vi "update_param_expSD.vi"(3 "cluster in":T1={"Kinetics"=[], "Spectrum"=[], "Experiments groups"=[], "GRAPH EXPERIMENTAL DATA"=[], "error out"={"status"=FALSE, "code"=0, "source"=""}, "group"=0, "exp selected"=0, "# exp"=0, "kinetics plot names"=[], "spectra plot names"=[], "FromToWave"={"FromWave"=0.0, "ToWave"=0.0}, "Laser shutter task"="", "Accelerator task"="", "Motor task"="", "GRAPH EXPERIMENTAL DATA ref"=refnum, "timedelays"=[0.0, 0.0, 0.0, 0.0, 0.0, 0.0, 0.0, 0.06019061100911815, 0.0521779104562645, 0.045231877429679615, 0.03921051490799832, 0.033990728811568754, 0.029465811603150715, 0.025543260876973825, 0.02214288834180205, 0.01919518054014414, 0.016639877791965713, 0.014424742312398925, 0.012504490320209958, 0.010839866306230088, 0.009396840537117498, 0.008145913389103785, 0.00706151229029317, 0.006121468943269439, 0.005306566140927374, 0.004600144911132549, 0.003987763959109073, 0.0034569044455719407, 0.00299671406541447, 0.0025977851951783253, 0.0022519625739982996, 0.00195217658646366, 0.0016922987392150965, 0.0014670163768006634, 0.0012717240756200802, 0.0011024294957352762, 0.0009556717658856477, 0.0008284507332614981, 0.0007181656316962257, 0.0006225619144775864, 0.0005396851648867825, 0.00046784114226338394, 0.0004055611468220084, 0.0003515719951773376, 0.00030476999279031153, 0.00026419837125694315, 0.00022902772919263772, 0.0001985390768670671, 0.0001721091379728629, 0.00014919760805372974, 0.00012933610911736794], "wavelengths"=[0.0, 0.0, 0.0, 0.0, 0.0, 0.0, 0.0, 0.06019061100911815, 0.0521779104562645, 0.045231877429679615, 0.03921051490799832, 0.033990728811568754, 0.029465811603150715, 0.025543260876973825, 0.02214288834180205, 0.01919518054014414, 0.016639877791965713, 0.014424742312398925, 0.012504490320209958, 0.010839866306230088, 0.009396840537117498, 0.008145913389103785, 0.00706151229029317, 0.006121468943269439, 0.005306566140927374, 0.004600144911132549, 0.003987763959109073, 0.0034569044455719407, 0.00299671406541447, 0.0025977851951783253, 0.0022519625739982996, 0.00195217658646366, 0.0016922987392150965, 0.0014670163768006634, 0.0012717240756200802, 0.0011024294957352762, 0.0009556717658856477, 0.0008284507332614981, 0.0007181656316962257, 0.0006225619144775864, 0.0005396851648867825, 0.00046784114226338394, 0.0004055611468220084, 0.0003515719951773376, 0.00030476999279031153, 0.00026419837125694315, 0.00022902772919263772, 0.0001985390768670671, 0.0001721091379728629, 0.00014919760805372974, 0.00012933610911736794], "Experiment"=refnum, "Commentaires exp"=refnum, "FromToDelay"={"FromDelay"=0.0, "ToDelay"=0.0}}) -> (5 "Real delay time, ps":dbl=3790.0, 6 "numberpoints, ps":i32, 7 "deltaTlast":dbl, 8 "# current":i32, 9 "Delay0,ps":dbl=-200.0, 10 "cluster out":T1={"Kinetics"=[], "Spectrum"=[], "Experiments groups"=[], "GRAPH EXPERIMENTAL DATA"=[], "error out"={"status"=FALSE, "code"=0, "source"=""}, "group"=0, "exp selected"=0, "# exp"=0, "kinetics plot names"=[], "spectra plot names"=[], "FromToWave"={"FromWave"=0.0, "ToWave"=0.0}, "Laser shutter task"="", "Accelerator task"="", "Motor task"="", "GRAPH EXPERIMENTAL DATA ref"=refnum, "timedelays"=[0.0, 0.0, 0.0, 0.0, 0.0, 0.0, 0.0, 0.06019061100911815, 0.0521779104562645, 0.045231877429679615, 0.03921051490799832, 0.033990728811568754, 0.029465811603150715, 0.025543260876973825, 0.02214288834180205, 0.01919518054014414, 0.016639877791965713, 0.014424742312398925, 0.012504490320209958, 0.010839866306230088, 0.009396840537117498, 0.008145913389103785, 0.00706151229029317, 0.006121468943269439, 0.005306566140927374, 0.004600144911132549, 0.003987763959109073, 0.0034569044455719407, 0.00299671406541447, 0.0025977851951783253, 0.0022519625739982996, 0.00195217658646366, 0.0016922987392150965, 0.0014670163768006634, 0.0012717240756200802, 0.0011024294957352762, 0.0009556717658856477, 0.0008284507332614981, 0.0007181656316962257, 0.0006225619144775864, 0.0005396851648867825, 0.00046784114226338394, 0.0004055611468220084, 0.0003515719951773376, 0.00030476999279031153, 0.00026419837125694315, 0.00022902772919263772, 0.0001985390768670671, 0.0001721091379728629, 0.00014919760805372974, 0.00012933610911736794], "wavelengths"=[0.0, 0.0, 0.0, 0.0, 0.0, 0.0, 0.0, 0.06019061100911815, 0.0521779104562645, 0.045231877429679615, 0.03921051490799832, 0.033990728811568754, 0.029465811603150715, 0.025543260876973825, 0.02214288834180205, 0.01919518054014414, 0.016639877791965713, 0.014424742312398925, 0.012504490320209958, 0.010839866306230088, 0.009396840537117498, 0.008145913389103785, 0.00706151229029317, 0.006121468943269439, 0.005306566140927374, 0.004600144911132549, 0.003987763959109073, 0.0034569044455719407, 0.00299671406541447, 0.0025977851951783253, 0.0022519625739982996, 0.00195217658646366, 0.0016922987392150965, 0.0014670163768006634, 0.0012717240756200802, 0.0011024294957352762, 0.0009556717658856477, 0.0008284507332614981, 0.0007181656316962257, 0.0006225619144775864, 0.0005396851648867825, 0.00046784114226338394, 0.0004055611468220084, 0.0003515719951773376, 0.00030476999279031153, 0.00026419837125694315, 0.00022902772919263772, 0.0001985390768670671, 0.0001721091379728629, 0.00014919760805372974, 0.00012933610911736794], "Experiment"=refnum, "Commentaires exp"=refnum, "FromToDelay"={"FromDelay"=0.0, "ToDelay"=0.0}})   [LabVIEW 2015]
uses:
  controls/control-cluster.ctl
  Classes/Experiments_group.lvclass
  Classes/Experiment.lvclass
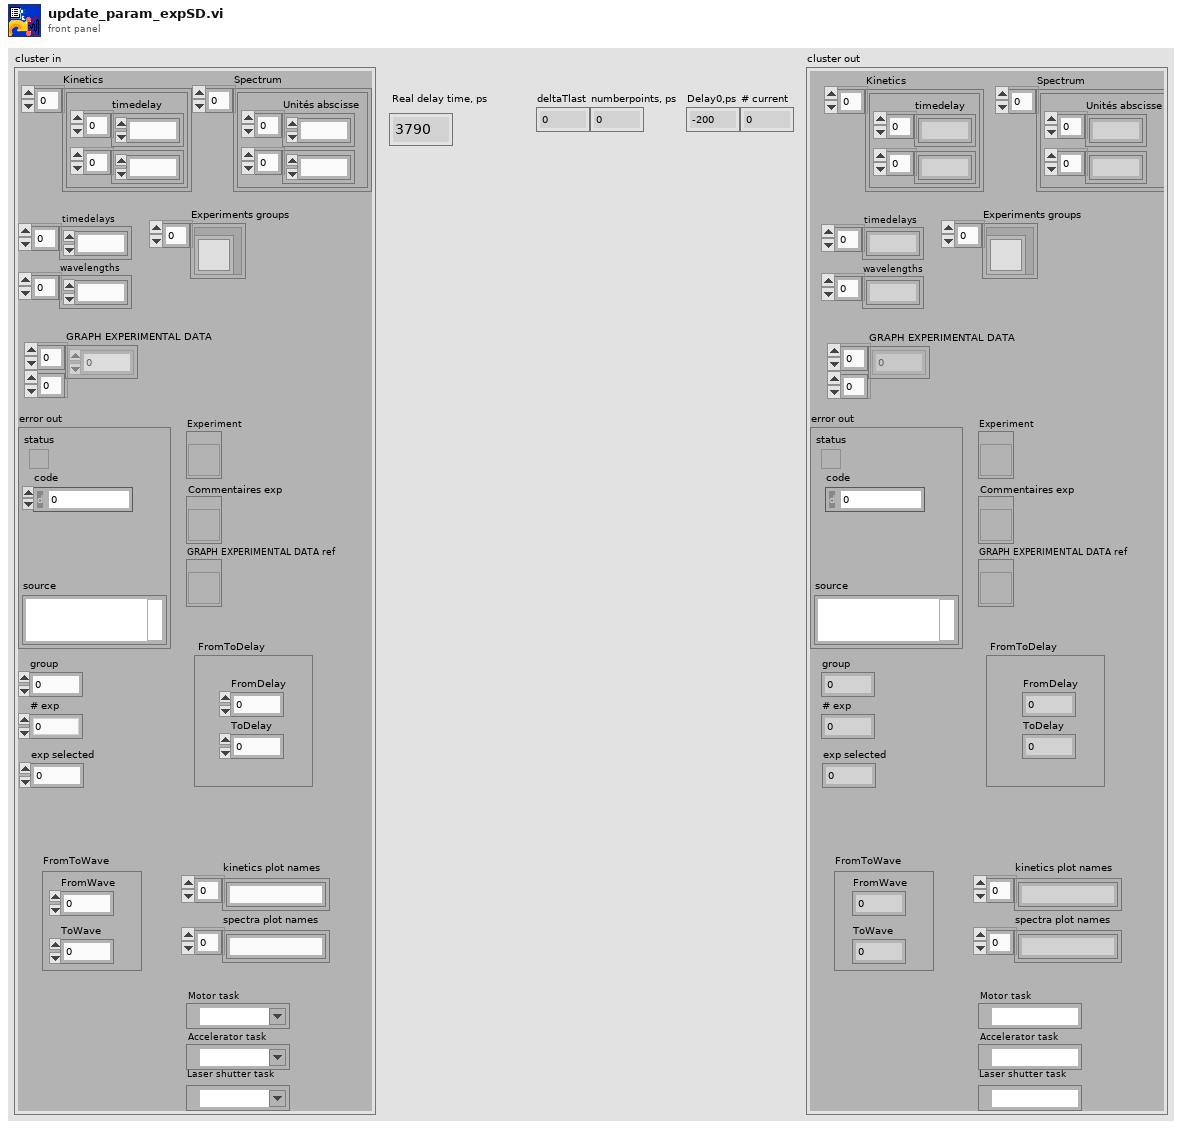
[diagram p1: front panel]
types:
  T1 = typedef "control-cluster.ctl" = cluster{"Kinetics":cluster{"timedelay":dbl[], dbl[]}[], "Spectrum":cluster{"Unités abscisse":dbl[], dbl[]}[], "Experiments groups":refnum<class "Experiments_group.lvclass">[], "GRAPH EXPERIMENTAL DATA":dbl[][], "error out":errorcluster, "group":i32, "exp selected":i32, "# exp":i32, "kinetics plot names":string[], "spectra plot names":string[], "FromToWave":cluster{"FromWave":dbl, "ToWave":dbl}, "Laser shutter task":refnum<k21>, "Accelerator task":refnum<k21>, "Motor task":refnum<k21>, "GRAPH EXPERIMENTAL DATA ref":refnum<vi>, "timedelays":dbl[], "wavelengths":dbl[], "Experiment":refnum<vi>, "Commentaires exp":refnum<vi>, "FromToDelay":cluster{"FromDelay":dbl, "ToDelay":dbl}}
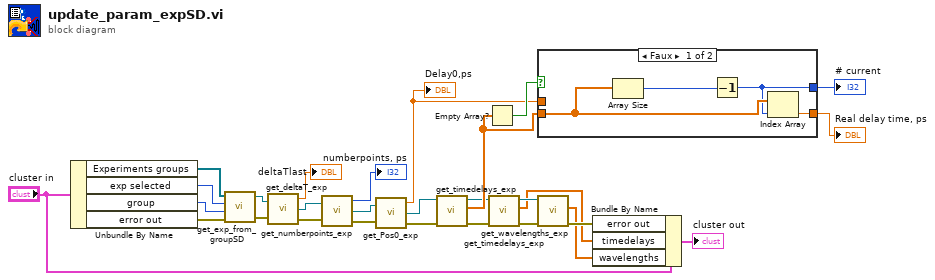
[diagram p0: block diagram]
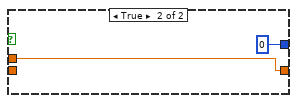
[diagram p2: hidden frame]
diagram:
  n1 = Unbundle By Name("cluster in") -> ("Experiments groups"=w14:refnum<class "Experiments_group.lvclass">[], "exp selected"=w15:i32, "group"=w16:i32, "error out"=w21:errorcluster)
  n2 = call "get_exp_from_groupSD.vi"("error in (no error)"=w21, "group"=w16, "exp selected"=w15, "Experiments groups"=w14) -> ("error out"=w20:errorcluster, "Experiment out"=w17:refnum<class "Experiment.lvclass">)  [unwired: 1 out]
  n3 = call-dynamic "get_deltaT_exp.vi"("Experiment.lvclass in"=w17, "error in (no error)"=w20) -> ("deltaTlast"=→"deltaTlast":dbl, "Experiment.lvclass out"=w18:refnum<class "Experiment.lvclass">, "error out"=w22:errorcluster)
  n4 = call-dynamic "get_numberpoints_exp.vi"("Experiment.lvclass in"=w18, "error in (no error)"=w22) -> ("numberpoints"=→"numberpoints, ps":i32, "Experiment.lvclass out"=w19:refnum<class "Experiment.lvclass">, "error out"=w23:errorcluster)
  n5 = call-dynamic "get_Pos0_exp.vi"("Experiment.lvclass in"=w19, "error in (no error)"=w23) -> ("Delay0,ps"=w11:dbl, "Experiment.lvclass out"=w27:refnum<class "Experiment.lvclass">, "error out"=w26:errorcluster)
  "Delay0,ps" <- w11
  n6 = call-dynamic "get_timedelays_exp.vi"("error in (no error)"=w26, "Experiment.lvclass in"=w27) -> ("error out"=w5:errorcluster, "timedelays"=w9:dbl[], "Experiment.lvclass out"=w7:refnum<class "Experiment.lvclass">)  [unwired: 7 in]
  n7 = Empty Array?(array=w9) -> (empty?=w12:bool)
  n8 = call-dynamic "get_timedelays_exp.vi"("error in (no error)"=w5, "Experiment.lvclass in"=w7) -> ("error out"=w4:errorcluster, "timedelays"=w2:dbl[], "Experiment.lvclass out"=w6:refnum<class "Experiment.lvclass">)  [unwired: 7 in]
  n9 = case shown="Faux" w12 {
    tunnel: w11 -> [_ w34]
    tunnel: [w32 w34] -> w10
    tunnel: w9 -> [w31 _]
    tunnel: [w29 0 ("x")] -> w8
    frame False {
      n10 = Array Size(array=w31) -> (size(s)=w30:i32)
      n11 = Decrement(x=w30) -> (x-1=w29:i32)
      n12 = Index Array(array=w31, index=w29) -> (element=w32:dbl)
    }
    frame True {
    }
  }
  "Real delay time, ps" <- w10
  "# current" <- w8
  n13 = call-dynamic "get_wavelengths_exp.vi"("error in (no error)"=w4, "Experiment.lvclass in"=w6) -> ("error out"=w3:errorcluster, "wavelengths"=w1:dbl[])  [unwired: 7 in, 1 out]
  n14 = Bundle By Name(cluster="cluster in", "error out"=w3, "timedelays"=w2, "wavelengths"=w1) -> (→"cluster out":T1)
